vi "Typhon_Software-Ignitor.vi"() -> ()   [LabVIEW 2020]
uses:
  <vilib>/DAQmx/write.llb/DAQmx Write (Digital 1D Bool 1Chan 1Samp).vi
  <vilib>/DAQmx/create/channels.llb/DAQmx Create Channel (DO-Digital Output).vi
  <vilib>/DAQmx/miscellaneous.llb/DAQmx Fill In Error Info.vi
panel:
  out "E-Match":bool
  out "N2-CH4":bool
  out "N2-GOX":bool
  out "CH4  Isolation":bool
  out "CH4  Upper":bool
  out "GOX Isolation":bool
  out "GOX Upper":bool
  out "State":i32
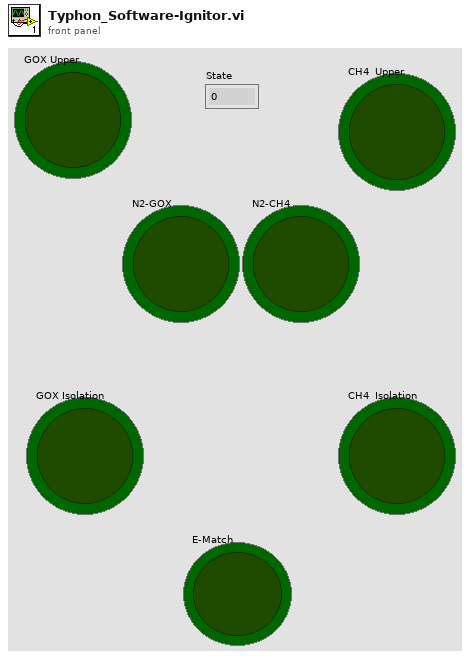
[diagram p1: front panel]
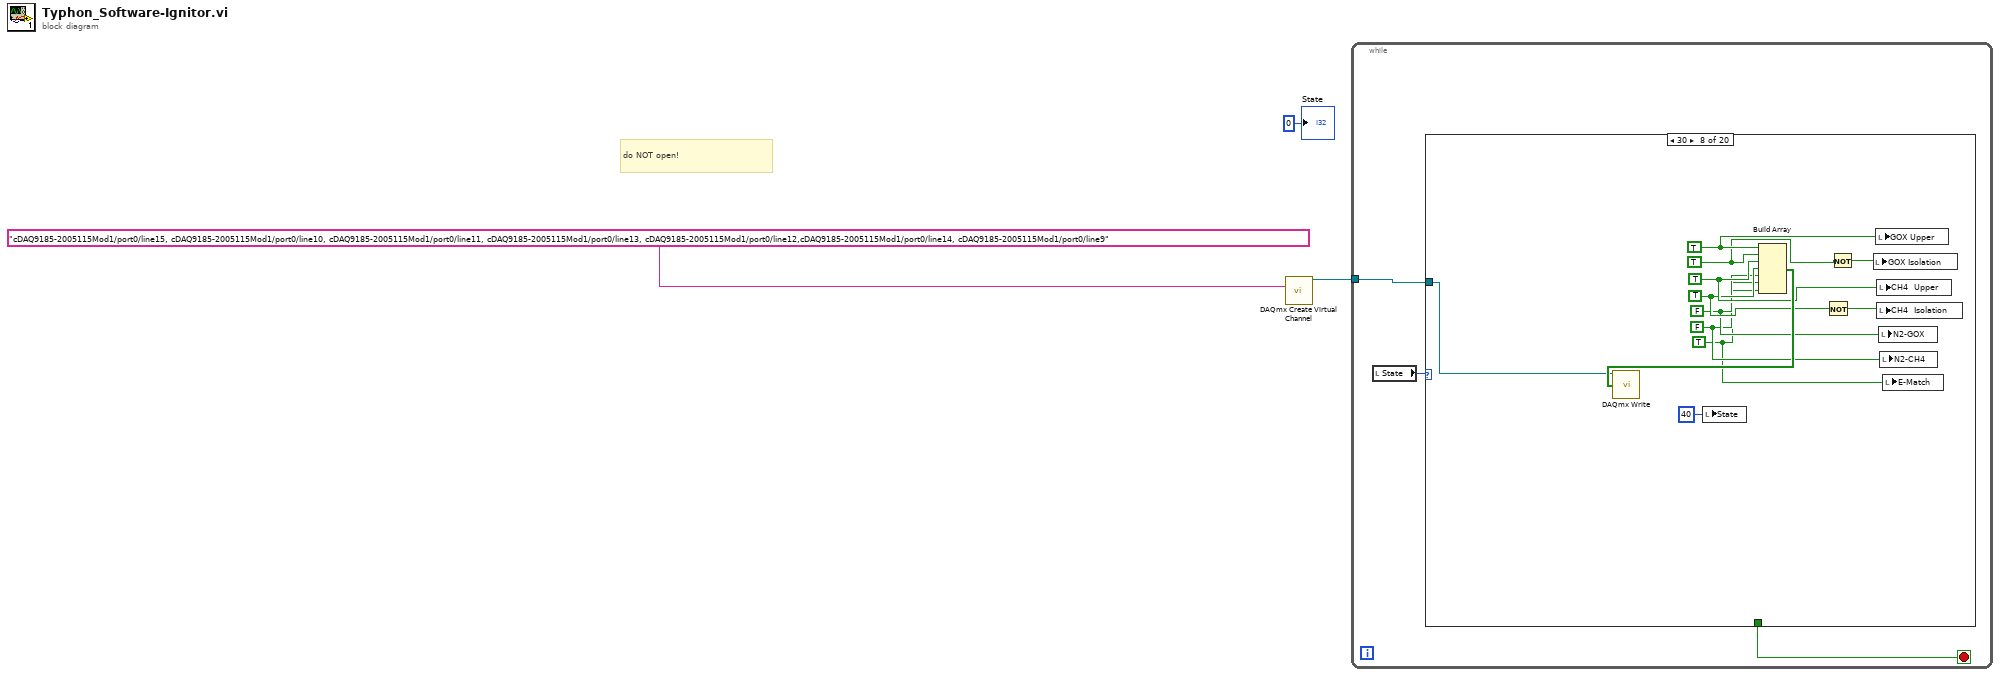
[diagram p0: block diagram]
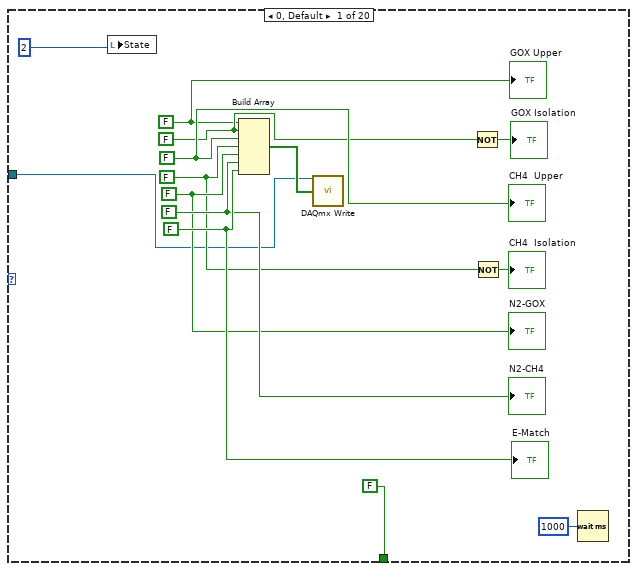
[diagram p2: hidden frame]
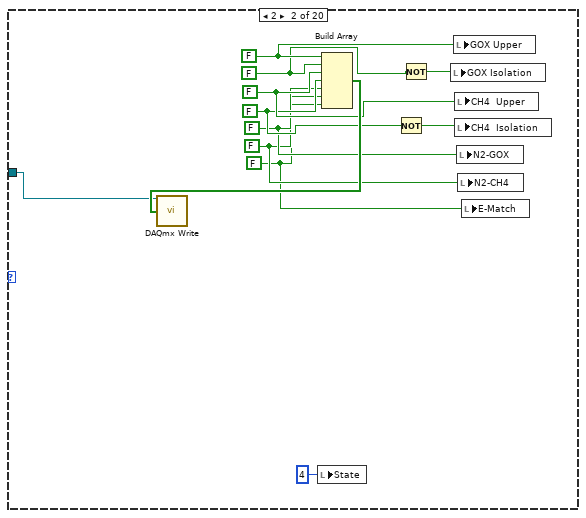
[diagram p3: hidden frame]
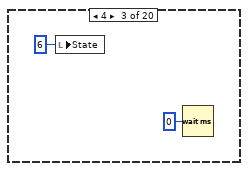
[diagram p4: hidden frame]
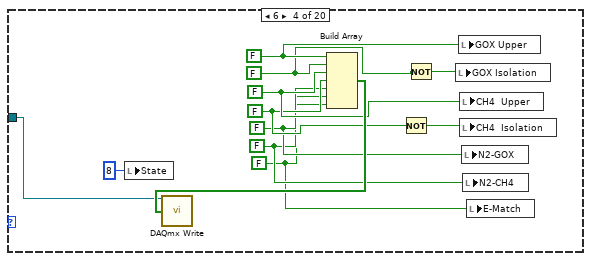
[diagram p5: hidden frame]
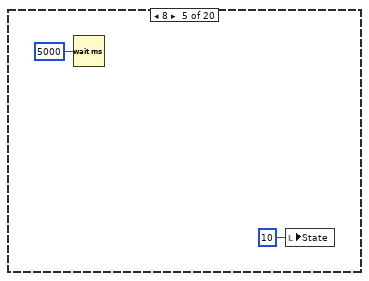
[diagram p6: hidden frame]
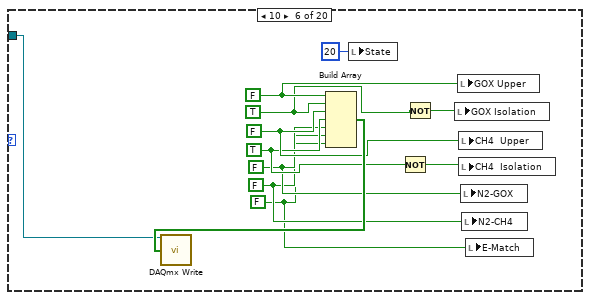
[diagram p7: hidden frame]
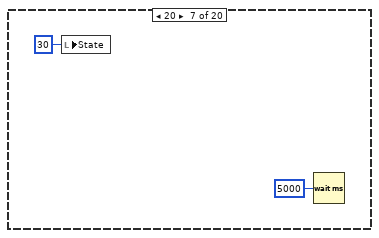
[diagram p8: hidden frame]
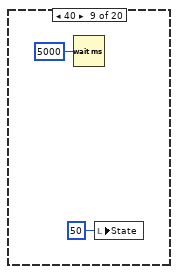
[diagram p9: hidden frame]
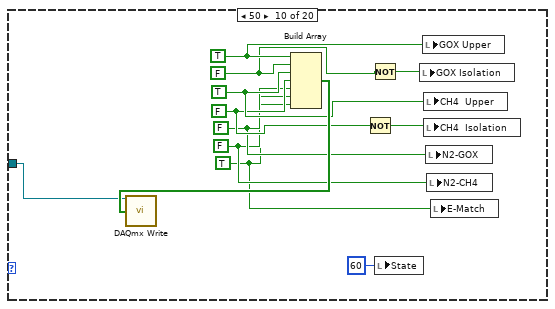
[diagram p10: hidden frame]
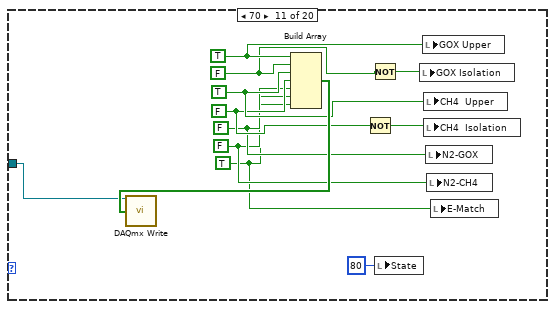
[diagram p11: hidden frame]
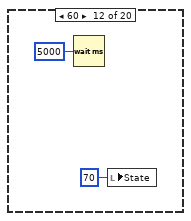
[diagram p12: hidden frame]
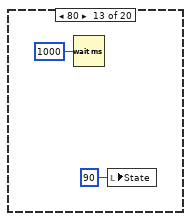
[diagram p13: hidden frame]
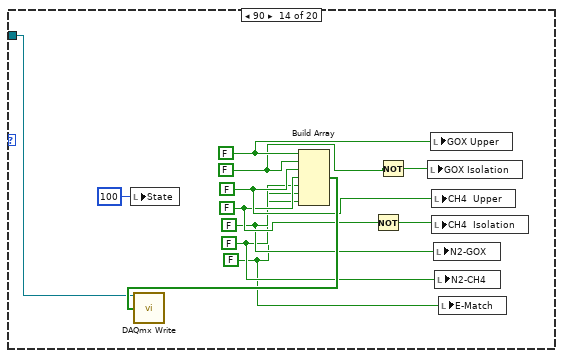
[diagram p14: hidden frame]
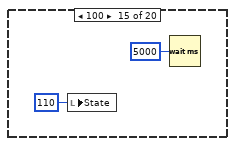
[diagram p15: hidden frame]
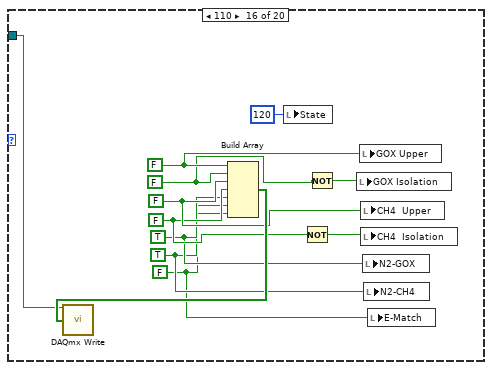
[diagram p16: hidden frame]
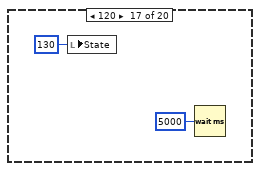
[diagram p17: hidden frame]
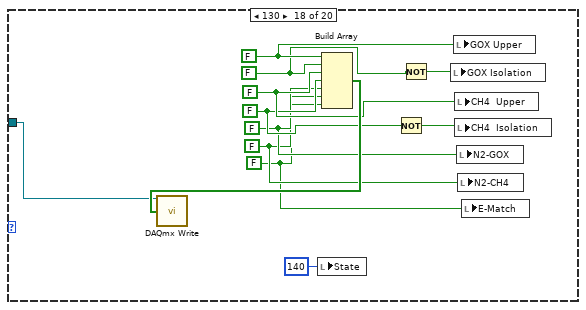
[diagram p18: hidden frame]
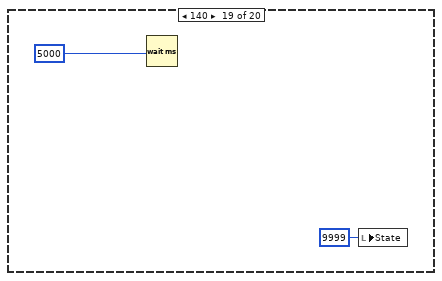
[diagram p19: hidden frame]
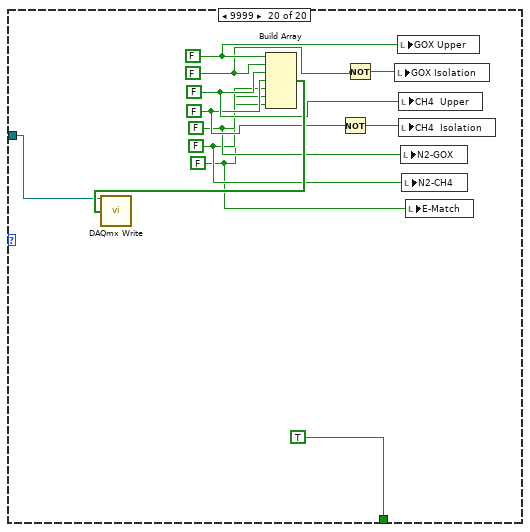
[diagram p20: hidden frame]
diagram:
  # "do NOT open!"
  n1 = call-poly <vilib>:"DAQmx Create Virtual Channel.vi"("lines"=tag "cDAQ9185-2005115Mod1/port0/line15, cDAQ9185-2005115Mod1/port0/line10, cDAQ9185-2005115Mod1/port0/line11, cDAQ9185-2005115Mod1/port0/line13, cDAQ9185-2005115Mod1/port0/line12,cDAQ9185-2005115Mod1/port0/line14, cDAQ9185-2005115Mod1/port0/line9") -> ("task out"=w1:refnum<k21>)  [unwired: 13 in, 1 out]
  n2 = while {
    tunnel: w1 -> [w5]
    stop <- w4 stop-if-true
    n3 = local read "State"() -> (w6:i32)
    n4 = case shown="30" w6 {
      tunnel: [FALSE _ _ _ _ _ _ _ _ _ _ _ _ _ _ _ _ _ _ TRUE] -> w4
      tunnel: w5 -> [w7 w21 _ w35 _ w49 _ w63 _ w77 w89 _ _ w105 _ w119 _ w133 _ w147]
      frame 0, Default {
        w14 = FALSE ("element")
        w13 = FALSE ("element")
        w12 = FALSE ("element")
        w11 = FALSE ("element")
        w10 = FALSE ("element")
        w9 = FALSE
        w8 = FALSE
        n5 = local write "State"(2 ("State")) -> ()
        n6 = Build Array(w8, w9, w10, w11, w12, w13, w14) -> (w15:bool[])
        n7 = call-poly <vilib>:"DAQmx Write.vi"("task/channels in"=w7, "data"=w15) -> ()  [unwired: 11 in, 3 out]
        n8 = Not(x=w9) -> (.not. x?=→"GOX Isolation":bool)
        n9 = Not(x=w11) -> (.not. x?=→"CH4  Isolation":bool)
        n10 = Wait (ms)(milliseconds to wait=u32 1000) -> ()  [unwired: 1 out]
        "GOX Upper" <- w8
        "CH4  Upper" <- w10
        "N2-GOX" <- w12
        "N2-CH4" <- w13
        "E-Match" <- w14
      }
      frame 2 {
        w22 = FALSE ("element")
        w23 = FALSE ("element")
        w24 = FALSE ("element")
        w25 = FALSE ("element")
        w26 = FALSE ("element")
        w27 = FALSE
        w28 = FALSE
        n11 = local write "State"(4 ("State")) -> ()
        n12 = Build Array(w28, w27, w26, w25, w24, w23, w22) -> (w31:bool[])
        n13 = call-poly <vilib>:"DAQmx Write.vi"("task/channels in"=w21, "data"=w31) -> ()  [unwired: 11 in, 3 out]
        n14 = Not(x=w25) -> (.not. x?=w30:bool)
        n15 = Not(x=w27) -> (.not. x?=w29:bool)
        n16 = local write "GOX Isolation"(w29) -> ()
        n17 = local write "GOX Upper"(w28) -> ()
        n18 = local write "CH4  Upper"(w26) -> ()
        n19 = local write "CH4  Isolation"(w30) -> ()
        n20 = local write "N2-GOX"(w24) -> ()
        n21 = local write "N2-CH4"(w23) -> ()
        n22 = local write "E-Match"(w22) -> ()
      }
      frame 4 {
        n23 = local write "State"(6 ("State")) -> ()
        n24 = Wait (ms)(milliseconds to wait=u32 0) -> ()  [unwired: 1 out]
      }
      frame 6 {
        w36 = FALSE ("element")
        w37 = FALSE ("element")
        w38 = FALSE ("element")
        w39 = FALSE ("element")
        w40 = FALSE ("element")
        w41 = FALSE
        w42 = FALSE
        n25 = local write "State"(8 ("State")) -> ()
        n26 = Build Array(w42, w41, w40, w39, w38, w37, w36) -> (w45:bool[])
        n27 = call-poly <vilib>:"DAQmx Write.vi"("task/channels in"=w35, "data"=w45) -> ()  [unwired: 11 in, 3 out]
        n28 = Not(x=w39) -> (.not. x?=w44:bool)
        n29 = Not(x=w41) -> (.not. x?=w43:bool)
        n30 = local write "GOX Isolation"(w43) -> ()
        n31 = local write "GOX Upper"(w42) -> ()
        n32 = local write "CH4  Upper"(w40) -> ()
        n33 = local write "CH4  Isolation"(w44) -> ()
        n34 = local write "N2-GOX"(w38) -> ()
        n35 = local write "N2-CH4"(w37) -> ()
        n36 = local write "E-Match"(w36) -> ()
      }
      frame 8 {
        n37 = Wait (ms)(milliseconds to wait=u32 5000) -> ()  [unwired: 1 out]
        n38 = local write "State"(10 ("State")) -> ()
      }
      frame 10 {
        w50 = FALSE ("element")
        w51 = FALSE ("element")
        w52 = FALSE ("element")
        w53 = TRUE ("element")
        w54 = FALSE ("element")
        w55 = TRUE
        w56 = FALSE
        n39 = Build Array(w56, w55, w54, w53, w52, w51, w50) -> (w59:bool[])
        n40 = call-poly <vilib>:"DAQmx Write.vi"("task/channels in"=w49, "data"=w59) -> ()  [unwired: 11 in, 3 out]
        n41 = local write "State"(20 ("State")) -> ()
        n42 = Not(x=w53) -> (.not. x?=w58:bool)
        n43 = Not(x=w55) -> (.not. x?=w57:bool)
        n44 = local write "GOX Isolation"(w57) -> ()
        n45 = local write "GOX Upper"(w56) -> ()
        n46 = local write "CH4  Upper"(w54) -> ()
        n47 = local write "CH4  Isolation"(w58) -> ()
        n48 = local write "N2-GOX"(w52) -> ()
        n49 = local write "N2-CH4"(w51) -> ()
        n50 = local write "E-Match"(w50) -> ()
      }
      frame 20 {
        n51 = local write "State"(30 ("State")) -> ()
        n52 = Wait (ms)(milliseconds to wait=u32 5000) -> ()  [unwired: 1 out]
      }
      frame 30 {
        w64 = TRUE ("element")
        w65 = FALSE ("element")
        w66 = FALSE ("element")
        w67 = TRUE ("element")
        w68 = TRUE ("element")
        w69 = TRUE
        w70 = TRUE
        n53 = local write "State"(40 ("State")) -> ()
        n54 = Build Array(w70, w69, w68, w67, w66, w65, w64) -> (w73:bool[])
        n55 = call-poly <vilib>:"DAQmx Write.vi"("task/channels in"=w63, "data"=w73) -> ()  [unwired: 11 in, 3 out]
        n56 = Not(x=w67) -> (.not. x?=w72:bool)
        n57 = Not(x=w69) -> (.not. x?=w71:bool)
        n58 = local write "GOX Isolation"(w71) -> ()
        n59 = local write "GOX Upper"(w70) -> ()
        n60 = local write "CH4  Upper"(w68) -> ()
        n61 = local write "CH4  Isolation"(w72) -> ()
        n62 = local write "N2-GOX"(w66) -> ()
        n63 = local write "N2-CH4"(w65) -> ()
        n64 = local write "E-Match"(w64) -> ()
      }
      frame 40 {
        n65 = Wait (ms)(milliseconds to wait=u32 5000) -> ()  [unwired: 1 out]
        n66 = local write "State"(50 ("State")) -> ()
      }
      frame 50 {
        w78 = TRUE ("element")
        w79 = FALSE ("element")
        w80 = FALSE ("element")
        w81 = FALSE ("element")
        w82 = TRUE ("element")
        w83 = FALSE
        w84 = TRUE
        n67 = Build Array(w84, w83, w82, w81, w80, w79, w78) -> (w87:bool[])
        n68 = call-poly <vilib>:"DAQmx Write.vi"("task/channels in"=w77, "data"=w87) -> ()  [unwired: 11 in, 3 out]
        n69 = Not(x=w81) -> (.not. x?=w86:bool)
        n70 = Not(x=w83) -> (.not. x?=w85:bool)
        n71 = local write "State"(60 ("State")) -> ()
        n72 = local write "GOX Isolation"(w85) -> ()
        n73 = local write "GOX Upper"(w84) -> ()
        n74 = local write "CH4  Upper"(w82) -> ()
        n75 = local write "CH4  Isolation"(w86) -> ()
        n76 = local write "N2-GOX"(w80) -> ()
        n77 = local write "N2-CH4"(w79) -> ()
        n78 = local write "E-Match"(w78) -> ()
      }
      frame 70 {
        w90 = TRUE ("element")
        w91 = FALSE ("element")
        w92 = FALSE ("element")
        w93 = FALSE ("element")
        w94 = TRUE ("element")
        w95 = FALSE
        w96 = TRUE
        n79 = Build Array(w96, w95, w94, w93, w92, w91, w90) -> (w99:bool[])
        n80 = call-poly <vilib>:"DAQmx Write.vi"("task/channels in"=w89, "data"=w99) -> ()  [unwired: 11 in, 3 out]
        n81 = Not(x=w93) -> (.not. x?=w98:bool)
        n82 = Not(x=w95) -> (.not. x?=w97:bool)
        n83 = local write "State"(80 ("State")) -> ()
        n84 = local write "GOX Isolation"(w97) -> ()
        n85 = local write "GOX Upper"(w96) -> ()
        n86 = local write "CH4  Upper"(w94) -> ()
        n87 = local write "CH4  Isolation"(w98) -> ()
        n88 = local write "N2-GOX"(w92) -> ()
        n89 = local write "N2-CH4"(w91) -> ()
        n90 = local write "E-Match"(w90) -> ()
      }
      frame 60 {
        n91 = Wait (ms)(milliseconds to wait=u32 5000) -> ()  [unwired: 1 out]
        n92 = local write "State"(70 ("State")) -> ()
      }
      frame 80 {
        n93 = Wait (ms)(milliseconds to wait=u32 1000) -> ()  [unwired: 1 out]
        n94 = local write "State"(90 ("State")) -> ()
      }
      frame 90 {
        w106 = FALSE ("element")
        w107 = FALSE ("element")
        w108 = FALSE ("element")
        w109 = FALSE ("element")
        w110 = FALSE ("element")
        w111 = FALSE
        w112 = FALSE
        n95 = local write "State"(100 ("State")) -> ()
        n96 = Build Array(w112, w111, w110, w109, w108, w107, w106) -> (w115:bool[])
        n97 = call-poly <vilib>:"DAQmx Write.vi"("task/channels in"=w105, "data"=w115) -> ()  [unwired: 11 in, 3 out]
        n98 = Not(x=w109) -> (.not. x?=w114:bool)
        n99 = Not(x=w111) -> (.not. x?=w113:bool)
        n100 = local write "GOX Isolation"(w113) -> ()
        n101 = local write "GOX Upper"(w112) -> ()
        n102 = local write "CH4  Upper"(w110) -> ()
        n103 = local write "CH4  Isolation"(w114) -> ()
        n104 = local write "N2-GOX"(w108) -> ()
        n105 = local write "N2-CH4"(w107) -> ()
        n106 = local write "E-Match"(w106) -> ()
      }
      frame 100 {
        n107 = local write "State"(110 ("State")) -> ()
        n108 = Wait (ms)(milliseconds to wait=u32 5000) -> ()  [unwired: 1 out]
      }
      frame 110 {
        w120 = FALSE ("element")
        w121 = TRUE ("element")
        w122 = TRUE ("element")
        w123 = FALSE ("element")
        w124 = FALSE ("element")
        w125 = FALSE
        w126 = FALSE
        n109 = Build Array(w126, w125, w124, w123, w122, w121, w120) -> (w129:bool[])
        n110 = call-poly <vilib>:"DAQmx Write.vi"("task/channels in"=w119, "data"=w129) -> ()  [unwired: 11 in, 3 out]
        n111 = local write "State"(120 ("State")) -> ()
        n112 = Not(x=w123) -> (.not. x?=w128:bool)
        n113 = Not(x=w125) -> (.not. x?=w127:bool)
        n114 = local write "GOX Isolation"(w127) -> ()
        n115 = local write "GOX Upper"(w126) -> ()
        n116 = local write "CH4  Upper"(w124) -> ()
        n117 = local write "CH4  Isolation"(w128) -> ()
        n118 = local write "N2-GOX"(w122) -> ()
        n119 = local write "N2-CH4"(w121) -> ()
        n120 = local write "E-Match"(w120) -> ()
      }
      frame 120 {
        n121 = local write "State"(130 ("State")) -> ()
        n122 = Wait (ms)(milliseconds to wait=u32 5000) -> ()  [unwired: 1 out]
      }
      frame 130 {
        w134 = FALSE ("element")
        w135 = FALSE ("element")
        w136 = FALSE ("element")
        w137 = FALSE ("element")
        w138 = FALSE ("element")
        w139 = FALSE
        w140 = FALSE
        n123 = local write "State"(140 ("State")) -> ()
        n124 = Build Array(w140, w139, w138, w137, w136, w135, w134) -> (w143:bool[])
        n125 = call-poly <vilib>:"DAQmx Write.vi"("task/channels in"=w133, "data"=w143) -> ()  [unwired: 11 in, 3 out]
        n126 = Not(x=w137) -> (.not. x?=w142:bool)
        n127 = Not(x=w139) -> (.not. x?=w141:bool)
        n128 = local write "GOX Isolation"(w141) -> ()
        n129 = local write "GOX Upper"(w140) -> ()
        n130 = local write "CH4  Upper"(w138) -> ()
        n131 = local write "CH4  Isolation"(w142) -> ()
        n132 = local write "N2-GOX"(w136) -> ()
        n133 = local write "N2-CH4"(w135) -> ()
        n134 = local write "E-Match"(w134) -> ()
      }
      frame 140 {
        n135 = Wait (ms)(milliseconds to wait=u32 5000) -> ()  [unwired: 1 out]
        n136 = local write "State"(9999 ("State")) -> ()
      }
      frame 9999 {
        w148 = FALSE ("element")
        w149 = FALSE ("element")
        w150 = FALSE ("element")
        w151 = FALSE ("element")
        w152 = FALSE ("element")
        w153 = FALSE
        w154 = FALSE
        n137 = Build Array(w154, w153, w152, w151, w150, w149, w148) -> (w157:bool[])
        n138 = call-poly <vilib>:"DAQmx Write.vi"("task/channels in"=w147, "data"=w157) -> ()  [unwired: 11 in, 3 out]
        n139 = Not(x=w151) -> (.not. x?=w156:bool)
        n140 = Not(x=w153) -> (.not. x?=w155:bool)
        n141 = local write "GOX Isolation"(w155) -> ()
        n142 = local write "GOX Upper"(w154) -> ()
        n143 = local write "CH4  Upper"(w152) -> ()
        n144 = local write "CH4  Isolation"(w156) -> ()
        n145 = local write "N2-GOX"(w150) -> ()
        n146 = local write "N2-CH4"(w149) -> ()
        n147 = local write "E-Match"(w148) -> ()
      }
    }
  }
  "State" <- 0 ("State")
